vi "Generate Rotated SICK Array.vi"(8 "error in (no error)":errorcluster, 10 "Close SICK":cluster{"x":dbl, "y":dbl}[](array[cluster])) -> (0 "error out":errorcluster, 2 "Rotated SICK Array":T1(array[cluster]))   [LabVIEW 2009]
uses:
  <vilib>/Analysis/Matrix/Datatypes/RealMatrix.ctl
  <vilib>/Analysis/baseanly.llb/Real A x B.vi
  <vilib>/Analysis/Matrix/NI_Matrix.lvlib
  <vilib>/Analysis/NI_AALBase.lvlib
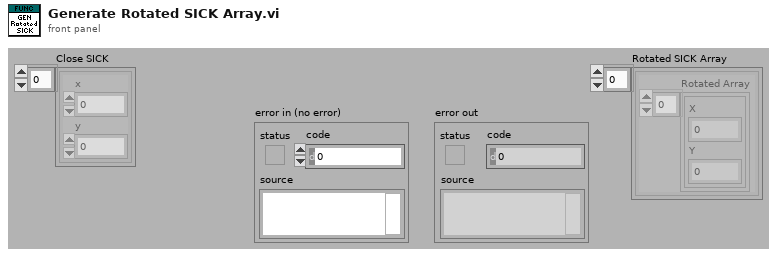
[diagram p1: front panel]
types:
  T1 = cluster{"Rotated Array":cluster{"X":dbl, "Y":dbl}[]}[]
  T2 = typedef "NI_Matrix.lvlib/RealMatrix.ctl" = dbl[][]
  T3 = cluster{"Rotated Array":cluster{"X":dbl, "Y":dbl}[]}
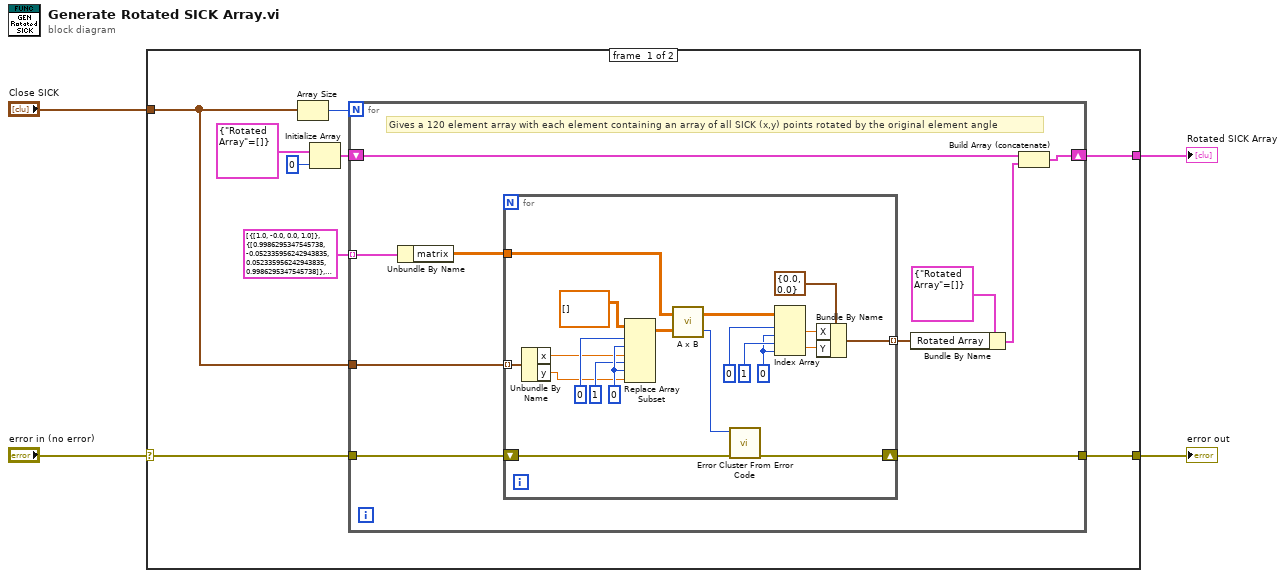
[diagram p0: block diagram]
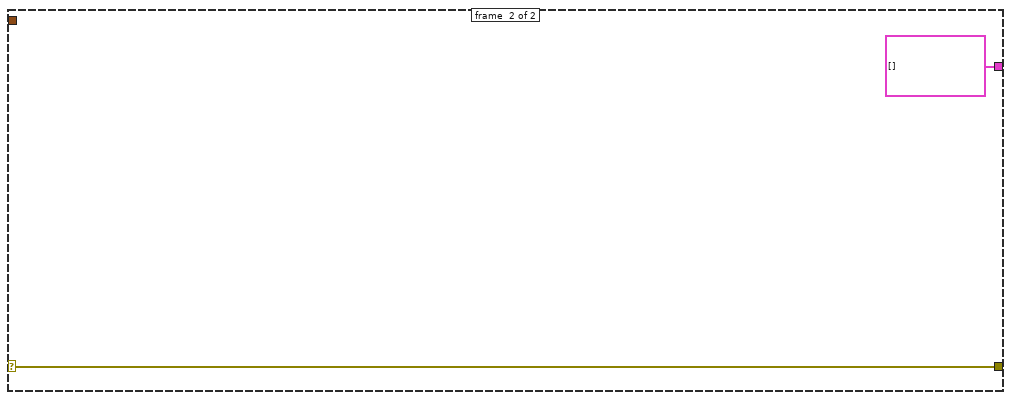
[diagram p2: hidden frame]
diagram:
  n1 = case shown="No Error" "error in (no error)" {
    selector: "error in (no error)" -> [w5 w45]
    tunnel: "Close SICK" -> [w8 _]
    tunnel: [w7 w45] -> w3
    tunnel: [w6 T1 []] -> w2
    frame #0 {
      n2 = Array Size(array=w8) -> (size(s)=w9:i32)
      n3 = Initialize Array(T3 {"Rotated Array"=[]} ("Cluster"), 0 ("dimension size")) -> (w11:T1)
      n4 = for {
        N: w9 -> [_]
        shift-right: [w15] -> w6
        shift-left: w11 -> [w17]
        tunnel: cluster{"matrix":T2}[] [{"matrix"=[[1.0, -0.0], [0.0, 1.0]]}, {"matrix"=[[0.9986295347545738, -0.052335956242943835], [0.052335956242943835, 0.9986295347545738]]}, {"matrix"=[[0.9945218953682733, -0.10452846326765347], [0.10452846326765347, 0.9945218953682733]]}, {"matrix"=[[0.9876883405951378, -0.15643446504023087], [0.15643446504023087, 0.9876883405951378]]}, {"matrix"=[[0.9781476007338057, -0.20791169081775934], [0.20791169081775934, 0.9781476007338057]]}, {"matrix"=[[0.9659258262890683, -0.25881904510252074], [0.25881904510252074, 0.9659258262890683]]}, {"matrix"=[[0.9510565162951535, -0.3090169943749474], [0.3090169943749474, 0.9510565162951535]]}, {"matrix"=[[0.9335804264972017, -0.35836794954530027], [0.35836794954530027, 0.9335804264972017]]}, {"matrix"=[[0.9135454576426009, -0.4067366430758002], [0.4067366430758002, 0.9135454576426009]]}, {"matrix"=[[0.8910065241883679, -0.45399049973954675], [0.45399049973954675, 0.8910065241883679]]}, {"matrix"=[[0.8660254037844387, -0.49999999999999994], [0.49999999999999994, 0.8660254037844387]]}, {"matrix"=[[0.838670567945424, -0.5446390350150271], [0.5446390350150271, 0.838670567945424]]}, {"matrix"=[[0.8090169943749475, -0.5877852522924731], [0.5877852522924731, 0.8090169943749475]]}, {"matrix"=[[0.7771459614569709, -0.6293203910498374], [0.6293203910498374, 0.7771459614569709]]}, {"matrix"=[[0.7431448254773942, -0.6691306063588582], [0.6691306063588582, 0.7431448254773942]]}, {"matrix"=[[0.7071067811865476, -0.7071067811865475], [0.7071067811865475, 0.7071067811865476]]}, {"matrix"=[[0.6691306063588582, -0.7431448254773942], [0.7431448254773942, 0.6691306063588582]]}, {"matrix"=[[0.6293203910498375, -0.7771459614569709], [0.7771459614569709, 0.6293203910498375]]}, {"matrix"=[[0.5877852522924731, -0.8090169943749475], [0.8090169943749475, 0.5877852522924731]]}, {"matrix"=[[0.5446390350150271, -0.838670567945424], [0.838670567945424, 0.5446390350150271]]}, {"matrix"=[[0.5000000000000001, -0.8660254037844386], [0.8660254037844386, 0.5000000000000001]]}, {"matrix"=[[0.4539904997395468, -0.8910065241883678], [0.8910065241883678, 0.4539904997395468]]}, {"matrix"=[[0.4067366430758002, -0.9135454576426009], [0.9135454576426009, 0.4067366430758002]]}, {"matrix"=[[0.3583679495453004, -0.9335804264972017], [0.9335804264972017, 0.3583679495453004]]}, {"matrix"=[[0.30901699437494745, -0.9510565162951535], [0.9510565162951535, 0.30901699437494745]]}, {"matrix"=[[0.25881904510252074, -0.9659258262890683], [0.9659258262890683, 0.25881904510252074]]}, {"matrix"=[[0.20791169081775945, -0.9781476007338056], [0.9781476007338056, 0.20791169081775945]]}, {"matrix"=[[0.15643446504023092, -0.9876883405951378], [0.9876883405951378, 0.15643446504023092]]}, {"matrix"=[[0.10452846326765346, -0.9945218953682733], [0.9945218953682733, 0.10452846326765346]]}, {"matrix"=[[0.052335956242943966, -0.9986295347545738], [0.9986295347545738, 0.052335956242943966]]}, {"matrix"=[[6.123031769111886e-17, -1.0], [1.0, 6.123031769111886e-17]]}, {"matrix"=[[-0.05233595624294384, -0.9986295347545738], [0.9986295347545738, -0.05233595624294384]]}, {"matrix"=[[-0.10452846326765355, -0.9945218953682733], [0.9945218953682733, -0.10452846326765355]]}, {"matrix"=[[-0.1564344650402308, -0.9876883405951378], [0.9876883405951378, -0.1564344650402308]]}, {"matrix"=[[-0.20791169081775934, -0.9781476007338057], [0.9781476007338057, -0.20791169081775934]]}, {"matrix"=[[-0.25881904510252085, -0.9659258262890683], [0.9659258262890683, -0.25881904510252085]]}, {"matrix"=[[-0.30901699437494734, -0.9510565162951536], [0.9510565162951536, -0.30901699437494734]]}, {"matrix"=[[-0.35836794954530027, -0.9335804264972017], [0.9335804264972017, -0.35836794954530027]]}, {"matrix"=[[-0.40673664307580026, -0.9135454576426009], [0.9135454576426009, -0.40673664307580026]]}, {"matrix"=[[-0.4539904997395467, -0.8910065241883679], [0.8910065241883679, -0.4539904997395467]]}, {"matrix"=[[-0.4999999999999998, -0.8660254037844387], [0.8660254037844387, -0.4999999999999998]]}, {"matrix"=[[-0.5446390350150271, -0.8386705679454239], [0.8386705679454239, -0.5446390350150271]]}, {"matrix"=[[-0.587785252292473, -0.8090169943749475], [0.8090169943749475, -0.587785252292473]]}, {"matrix"=[[-0.6293203910498373, -0.777145961456971], [0.777145961456971, -0.6293203910498373]]}, {"matrix"=[[-0.6691306063588582, -0.7431448254773942], [0.7431448254773942, -0.6691306063588582]]}, {"matrix"=[[-0.7071067811865475, -0.7071067811865476], [0.7071067811865476, -0.7071067811865475]]}, {"matrix"=[[-0.743144825477394, -0.6691306063588583], [0.6691306063588583, -0.743144825477394]]}, {"matrix"=[[-0.7771459614569709, -0.6293203910498374], [0.6293203910498374, -0.7771459614569709]]}, {"matrix"=[[-0.8090169943749473, -0.5877852522924732], [0.5877852522924732, -0.8090169943749473]]}, {"matrix"=[[-0.8386705679454239, -0.5446390350150273], [0.5446390350150273, -0.8386705679454239]]}, {"matrix"=[[-0.8660254037844387, -0.49999999999999994], [0.49999999999999994, -0.8660254037844387]]}, {"matrix"=[[-0.8910065241883678, -0.45399049973954686], [0.45399049973954686, -0.8910065241883678]]}, {"matrix"=[[-0.9135454576426008, -0.40673664307580043], [0.40673664307580043, -0.9135454576426008]]}, {"matrix"=[[-0.9335804264972017, -0.3583679495453002], [0.3583679495453002, -0.9335804264972017]]}, {"matrix"=[[-0.9510565162951535, -0.3090169943749475], [0.3090169943749475, -0.9510565162951535]]}, {"matrix"=[[-0.9659258262890682, -0.258819045102521], [0.258819045102521, -0.9659258262890682]]}, {"matrix"=[[-0.9781476007338057, -0.20791169081775931], [0.20791169081775931, -0.9781476007338057]]}, {"matrix"=[[-0.9876883405951377, -0.15643446504023098], [0.15643446504023098, -0.9876883405951377]]}, {"matrix"=[[-0.9945218953682733, -0.10452846326765373], [0.10452846326765373, -0.9945218953682733]]}, {"matrix"=[[-0.9986295347545738, -0.05233595624294381], [0.05233595624294381, -0.9986295347545738]]}, {"matrix"=[[-1.0, -1.2246063538223773e-16], [1.2246063538223773e-16, -1.0]]}, {"matrix"=[[-0.9986295347545738, 0.052335956242943564], [-0.052335956242943564, -0.9986295347545738]]}, {"matrix"=[[-0.9945218953682733, 0.1045284632676535], [-0.1045284632676535, -0.9945218953682733]]}, {"matrix"=[[-0.9876883405951378, 0.15643446504023073], [-0.15643446504023073, -0.9876883405951378]]}, {"matrix"=[[-0.9781476007338056, 0.2079116908177595], [-0.2079116908177595, -0.9781476007338056]]}, {"matrix"=[[-0.9659258262890683, 0.2588190451025208], [-0.2588190451025208, -0.9659258262890683]]}, {"matrix"=[[-0.9510565162951536, 0.3090169943749473], [-0.3090169943749473, -0.9510565162951536]]}, {"matrix"=[[-0.9335804264972017, 0.35836794954530043], [-0.35836794954530043, -0.9335804264972017]]}, {"matrix"=[[-0.9135454576426009, 0.4067366430758002], [-0.4067366430758002, -0.9135454576426009]]}, {"matrix"=[[-0.8910065241883679, 0.4539904997395467], [-0.4539904997395467, -0.8910065241883679]]}, {"matrix"=[[-0.8660254037844386, 0.5000000000000001], [-0.5000000000000001, -0.8660254037844386]]}, {"matrix"=[[-0.838670567945424, 0.5446390350150271], [-0.5446390350150271, -0.838670567945424]]}, {"matrix"=[[-0.8090169943749476, 0.587785252292473], [-0.587785252292473, -0.8090169943749476]]}, {"matrix"=[[-0.7771459614569708, 0.6293203910498376], [-0.6293203910498376, -0.7771459614569708]]}, {"matrix"=[[-0.7431448254773942, 0.6691306063588582], [-0.6691306063588582, -0.7431448254773942]]}, {"matrix"=[[-0.7071067811865477, 0.7071067811865475], [-0.7071067811865475, -0.7071067811865477]]}, {"matrix"=[[-0.6691306063588581, 0.7431448254773944], [-0.7431448254773944, -0.6691306063588581]]}, {"matrix"=[[-0.6293203910498378, 0.7771459614569706], [-0.7771459614569706, -0.6293203910498378]]}, {"matrix"=[[-0.5877852522924732, 0.8090169943749473], [-0.8090169943749473, -0.5877852522924732]]}, {"matrix"=[[-0.544639035015027, 0.838670567945424], [-0.838670567945424, -0.544639035015027]]}, {"matrix"=[[-0.5000000000000004, 0.8660254037844384], [-0.8660254037844384, -0.5000000000000004]]}, {"matrix"=[[-0.4539904997395469, 0.8910065241883678], [-0.8910065241883678, -0.4539904997395469]]}, {"matrix"=[[-0.4067366430758001, 0.913545457642601], [-0.913545457642601, -0.4067366430758001]]}, {"matrix"=[[-0.3583679495453007, 0.9335804264972016], [-0.9335804264972016, -0.3583679495453007]]}, {"matrix"=[[-0.30901699437494756, 0.9510565162951535], [-0.9510565162951535, -0.30901699437494756]]}, {"matrix"=[[-0.25881904510252063, 0.9659258262890683], [-0.9659258262890683, -0.25881904510252063]]}, {"matrix"=[[-0.2079116908177598, 0.9781476007338056], [-0.9781476007338056, -0.2079116908177598]]}, {"matrix"=[[-0.15643446504023104, 0.9876883405951377], [-0.9876883405951377, -0.15643446504023104]]}, {"matrix"=[[-0.10452846326765336, 0.9945218953682734], [-0.9945218953682734, -0.10452846326765336]]}, {"matrix"=[[-0.052335956242944306, 0.9986295347545738], [-0.9986295347545738, -0.052335956242944306]]}, {"matrix"=[[-1.836909530733566e-16, 1.0], [-1.0, -1.836909530733566e-16]]}, {"matrix"=[[0.052335956242943946, 0.9986295347545738], [-0.9986295347545738, 0.052335956242943946]]}, {"matrix"=[[0.10452846326765299, 0.9945218953682734], [-0.9945218953682734, 0.10452846326765299]]}, {"matrix"=[[0.15643446504023067, 0.9876883405951378], [-0.9876883405951378, 0.15643446504023067]]}, {"matrix"=[[0.20791169081775943, 0.9781476007338056], [-0.9781476007338056, 0.20791169081775943]]}, {"matrix"=[[0.2588190451025203, 0.9659258262890684], [-0.9659258262890684, 0.2588190451025203]]}, {"matrix"=[[0.30901699437494723, 0.9510565162951536], [-0.9510565162951536, 0.30901699437494723]]}, {"matrix"=[[0.3583679495453004, 0.9335804264972017], [-0.9335804264972017, 0.3583679495453004]]}, {"matrix"=[[0.40673664307579976, 0.9135454576426011], [-0.9135454576426011, 0.40673664307579976]]}, {"matrix"=[[0.45399049973954664, 0.8910065241883679], [-0.8910065241883679, 0.45399049973954664]]}, {"matrix"=[[0.5000000000000001, 0.8660254037844386], [-0.8660254037844386, 0.5000000000000001]]}, {"matrix"=[[0.5446390350150266, 0.8386705679454243], [-0.8386705679454243, 0.5446390350150266]]}, {"matrix"=[[0.5877852522924729, 0.8090169943749476], [-0.8090169943749476, 0.5877852522924729]]}, {"matrix"=[[0.6293203910498375, 0.7771459614569708], [-0.7771459614569708, 0.6293203910498375]]}, {"matrix"=[[0.6691306063588578, 0.7431448254773946], [-0.7431448254773946, 0.6691306063588578]]}, {"matrix"=[[0.7071067811865474, 0.7071067811865477], [-0.7071067811865477, 0.7071067811865474]]}, {"matrix"=[[0.7431448254773942, 0.6691306063588581], [-0.6691306063588581, 0.7431448254773942]]}, {"matrix"=[[0.7771459614569706, 0.6293203910498378], [-0.6293203910498378, 0.7771459614569706]]}, {"matrix"=[[0.8090169943749473, 0.5877852522924734], [-0.5877852522924734, 0.8090169943749473]]}, {"matrix"=[[0.838670567945424, 0.544639035015027], [-0.544639035015027, 0.838670567945424]]}, {"matrix"=[[0.8660254037844384, 0.5000000000000004], [-0.5000000000000004, 0.8660254037844384]]}, {"matrix"=[[0.8910065241883678, 0.45399049973954697], [-0.45399049973954697, 0.8910065241883678]]}, {"matrix"=[[0.913545457642601, 0.40673664307580015], [-0.40673664307580015, 0.913545457642601]]}, {"matrix"=[[0.9335804264972015, 0.35836794954530077], [-0.35836794954530077, 0.9335804264972015]]}, {"matrix"=[[0.9510565162951535, 0.3090169943749476], [-0.3090169943749476, 0.9510565162951535]]}, {"matrix"=[[0.9659258262890683, 0.2588190451025207], [-0.2588190451025207, 0.9659258262890683]]}, {"matrix"=[[0.9781476007338056, 0.20791169081775987], [-0.20791169081775987, 0.9781476007338056]]}, {"matrix"=[[0.9876883405951377, 0.1564344650402311], [-0.1564344650402311, 0.9876883405951377]]}, {"matrix"=[[0.9945218953682733, 0.10452846326765342], [-0.10452846326765342, 0.9945218953682733]]}, {"matrix"=[[0.9986295347545738, 0.05233595624294437], [-0.05233595624294437, 0.9986295347545738]]}] ("Array") -> [w21] mode=indexing
        tunnel: w8 -> [w14]
        tunnel: w5 -> [w22]
        tunnel: [w23] -> w7
        # "Gives a 120 element array with each element containing an array of all SICK (x,y) points rotated by the original element angle"
        n5 = Unbundle By Name(w21) -> ("matrix"=w20:T2)
        n6 = for {
          shift-right: [w39] -> w23
          shift-left: w22 -> [w38]
          tunnel: w20 -> [w32]
          tunnel: [w30] -> w18 mode=indexing
          tunnel: w14 -> [w29] mode=indexing
          w36 = 0 ("index (col)")
          w41 = 0 ("index (col)")
          n7 = Unbundle By Name(w29) -> ("x"=w28:dbl, "y"=w27:dbl)
          n8 = Replace Array Subset(array=T2 [] ("matrix"), new element #1=w28, index (row) #1=0 ("disabled index (row)"), index (col) #1=w36, new element #2=w27, index (row) #2=1 ("disabled index (row)"), index (col) #2=w36) -> (w33:T2)
          n9 = call-poly <vilib>:"A x B.vi"("B"=w33, "A"=w32) -> ("error"=w40:i32, "A x B"=w24:T2)
          n10 = call <vilib>:"Error Cluster From Error Code.vi"("error in (no error)"=w38, "error code (0)"=w40) -> ("error out"=w39:errorcluster)  [unwired: 7 in]
          n11 = Index Array(array=w24, index (row) #1=0 ("disabled index (row)"), index (col) #1=w41, index (row) #2=1 ("disabled index (row)"), index (col) #2=w41) -> (element #1=w26:dbl, element #2=w25:dbl)
          n12 = Bundle By Name(cluster=cluster{"X":dbl, "Y":dbl} {"X"=0.0, "Y"=0.0} ("Cluster"), "X"=w26, "Y"=w25) -> (w30:cluster{"X":dbl, "Y":dbl})
        }
        n13 = Bundle By Name(cluster=T3 {"Rotated Array"=[]} ("Cluster"), "Rotated Array"=w18) -> (w16:T3)
        n14 = Build Array (concatenate)(w17, w16) -> (w15:T1)
      }
    }
    frame #1 {
    }
  }
  "error out" <- w3
  "Rotated SICK Array" <- w2
